vi "Call Cypher Driver.vi"(0 "Output Array":T1(array[cluster]), 1 "Offset":cluster{"X Offset":dbl, "Y Offset":dbl}, 5 "Distance Between Interpolated Points (nm)":dbl, 7 "Z Set Point (For Cypher AFM)":dbl, 9 "PID close":bool, 11 "Display the Wave (Cypher AFM)":bool, 12 "Image Size":cluster{"Width":dbl, "Height":dbl}) -> ()   [LabVIEW 2011]
doc: "This VI sends information in the correct format to the Cypher."
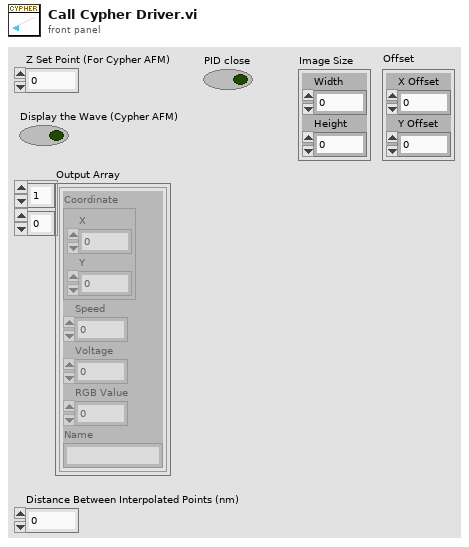
[diagram p1: front panel]
types:
  T1 = cluster{"Coordinate":cluster{"X":dbl, "Y":dbl}, "Speed":dbl, "Voltage":dbl, "RGB Value":i32, "Name":string}[][]
  T2 = cluster{"Coordinate":cluster{"X":dbl, "Y":dbl}, "Speed":dbl, "Voltage":dbl, "RGB Value":i32, "Name":string}
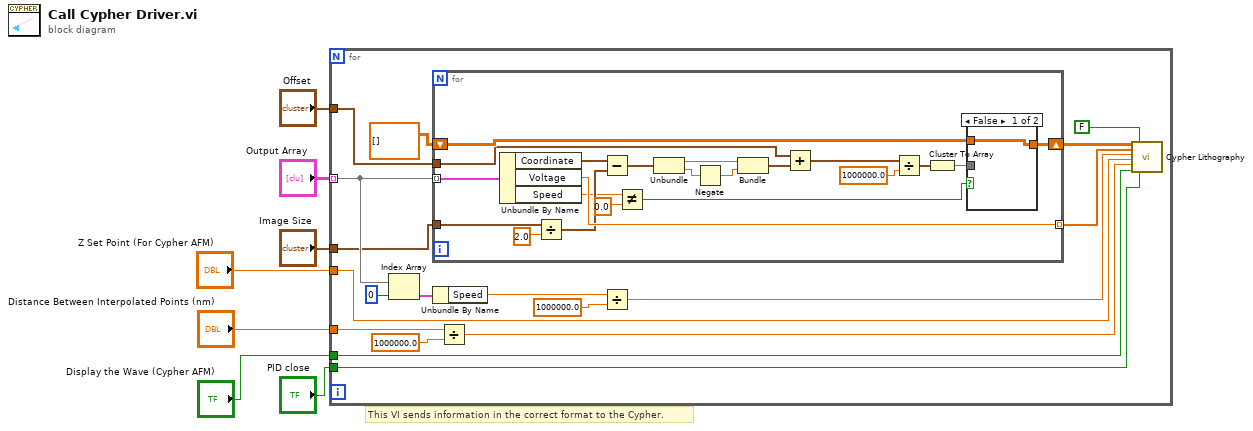
[diagram p0: block diagram]
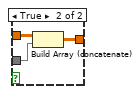
[diagram p2: hidden frame]
diagram:
  # "This VI sends information in the correct format to the Cypher."
  n1 = for {
    tunnel: "Distance Between Interpolated Points (nm)" -> [w12]
    tunnel: "Output Array" -> [w25] mode=indexing
    tunnel: "Z Set Point (For Cypher AFM)" -> [w20]
    tunnel: "Display the Wave (Cypher AFM)" -> [w19]
    tunnel: "PID close" -> [w18]
    tunnel: "Image Size" -> [w17]
    tunnel: "Offset" -> [w8]
    n2 = Index Array(array=w25, index=0) -> (element=w23:T2)
    n3 = for {
      tunnel: w25 -> [w46] mode=indexing
      tunnel: [w45] -> w21 mode=indexing
      tunnel: w17 -> [w43]
      shift-right: [w33] -> w10
      shift-left: dbl[][] [] -> [w32]
      tunnel: w8 -> [w26]
      n4 = Unbundle By Name(w46) -> ("Coordinate"=w40:cluster{"X":dbl, "Y":dbl}, "Voltage"=w45:dbl, "Speed"=w31:dbl)
      n5 = Divide(x=w43, y=2.0) -> (x/y=w39:cluster{"Width":dbl, "Height":dbl})
      n6 = Subtract(x=w40, y=w39) -> (x-y=w38:cluster{dbl, dbl})
      n7 = Not Equal?(x=w31, y=0.0) -> (x != y?=w29:bool)
      n8 = Unbundle(w38) -> (w35:dbl, w37:dbl)
      n9 = Negate(x=w37) -> (-x=w36:dbl)
      n10 = Bundle(w35, w36) -> (w28:cluster{dbl, dbl})  [unwired: 1 in]
      n11 = Add(x=w26, y=w28) -> (x+y=w27:cluster{dbl, dbl})
      n12 = Divide(x=w27, y=1000000.0) -> (x/y=w41:cluster{dbl, dbl})
      n13 = Cluster To Array(cluster=w41) -> (array=w34:dbl[])
      n14 = case shown="False" w29 {
        tunnel: w34 -> [_ w50]
        tunnel: [w47 w49] -> w33
        tunnel: w32 -> [w47 w48]
        frame False {
        }
        frame True {
          n15 = Build Array (concatenate)(w48, w50) -> (w49:dbl[][])
        }
      }
    }
    n16 = Unbundle By Name(w23) -> ("Speed"=w15:dbl)
    n17 = Divide(x=w12, y=1000000.0) -> (x/y=w11:dbl)
    n18 = Divide(x=w15, y=1000000.0) -> (x/y=w14:dbl)
    n19 = call "Cypher Lithography.vi"("Nodes on the line\n(  x      ,       y   )"=w10, "V"=w21, "Litho Speed"=w14, "Z SetPoint"=w20, "New nodes spacing"=w11, 5:w19, "Need interpolate new nodes?"=FALSE, "PID close"=w18) -> ()  [unwired: 12 in]
  }
